vi "Export dat - C-V.vi"(8 "Error In":errorcluster, 9 "Workspace":path, 11 "C-V measurement":T1 {"CV properties"."V range" items=["10mV"=0.01, "100mV"=0.1, "1V"=1.0, "10V"=10.0]; "CV properties"."I range" items=["100nA"=-7.0, "1µA"=-6.0, "10µA"=-5.0, "100µA"=-4.0, "1mA"=-3.0, "10mA"=-2.0]}) -> (0 "Error Out":errorcluster)   [LabVIEW 2019]
doc: "Handles export of a C-V measurement to a .dat file, displays a GUI window"
uses:
  Type defs/CV measurement Type Def.ctl
  Type defs/CV properties Type Def.ctl
  <vilib>/Utility/sysdir.llb/System Directory Type.ctl
  <vilib>/Utility/file.llb/Write Delimited Spreadsheet (string).vi
  <vilib>/Utility/file.llb/Write Delimited Spreadsheet (DBL).vi
panel:
  out "String":string
  in  "Path":path caption="Export file as:"
  in  "Export":bool
  in  "Cancel":bool
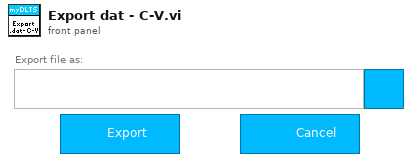
[diagram p1: front panel]
types:
  T1 = typedef "CV measurement Type Def.ctl" = cluster{"Name":string, "Comment":string, "Time":timestamp, "Folder":path, "CV properties":T2, "GUID":string}
  T2 = typedef "CV properties Type Def.ctl" = cluster{"T":dbl[unit], "Vstart":dbl[unit], "Vstop":dbl[unit], "Vpoints":dbl, "Precision":enum16{"Low (Fast)", "Normal", "High (Slow)"}, "Test signal":dbl[unit], "Auto I range":bool, "Test frequency":dbl[unit], "I range":dbl, "V range":dbl[unit], "Log mapping":bool, "Rel perm":dbl, "Area":dbl[unit]}
  T3 = enum32{"existing file", "new file", "new or existing file", "existing dir", "new dir", "new or existing dir", "existing file (use LLBs)", "new file (use LLBs)", "new or existing file (use LLBs)", "new or existing file or directory (use LLBs)", "existing dir (use LLBs)", "new dir (use LLBs)", "new or existing dir (use LLBs)", "existing file or dir", "new file or dir", "new or existing file or dir", "existing file or dir (use LLBs)", "new file or dir (use LLBs)"}
  T4 = typedef "System Directory Type.ctl" = i32
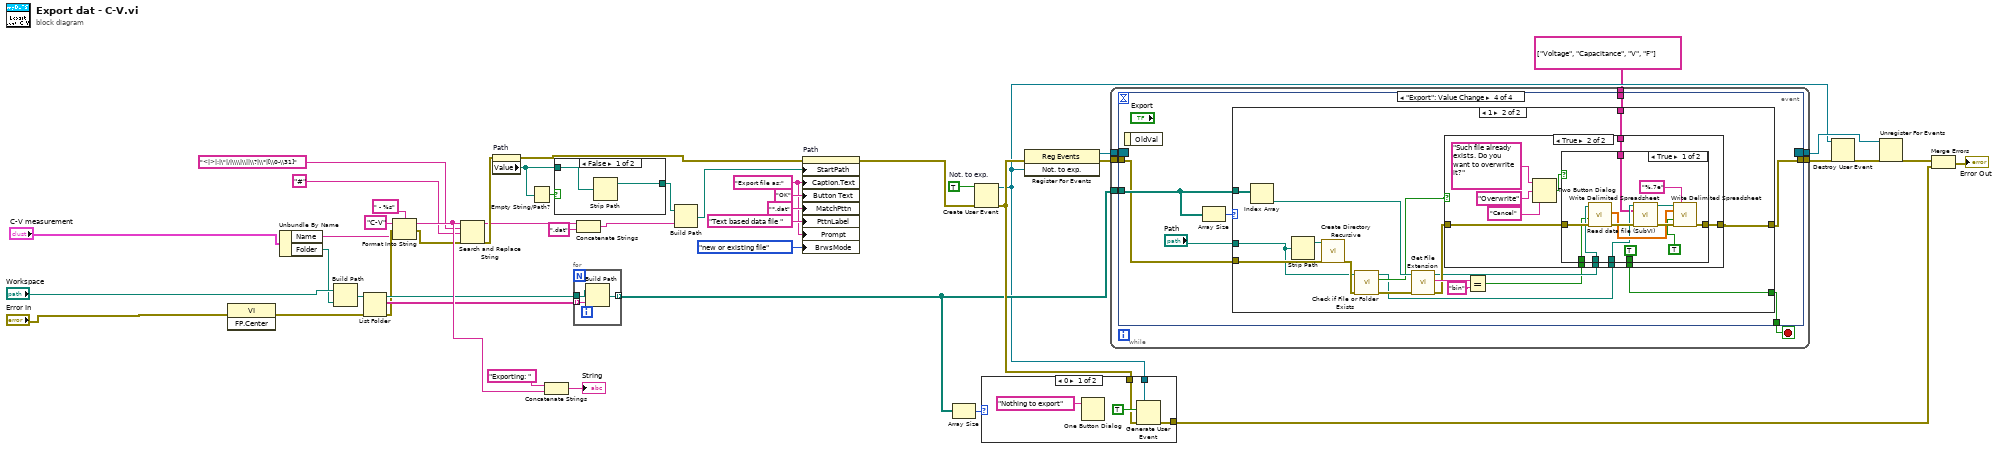
[diagram p0: block diagram]
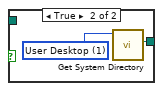
[diagram p2: hidden frame]
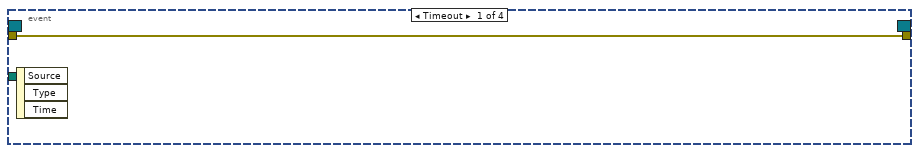
[diagram p4: hidden frame]
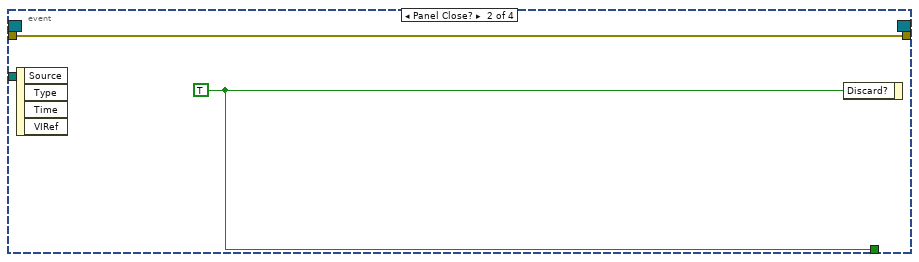
[diagram p5: hidden frame]
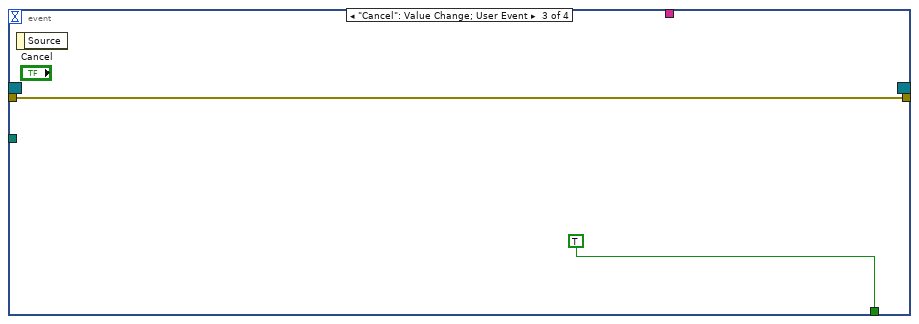
[diagram p6: hidden frame]
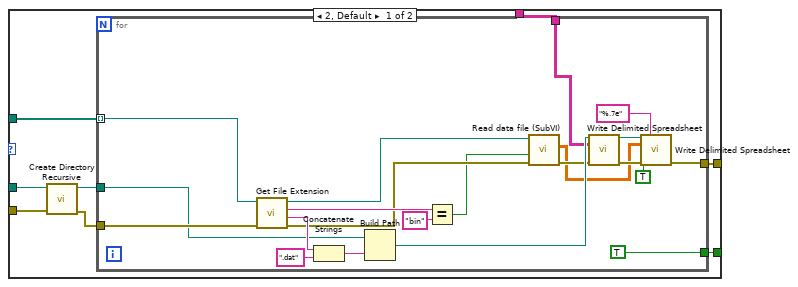
[diagram p7: hidden frame]
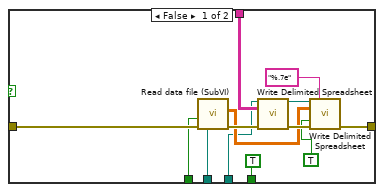
[diagram p8: hidden frame]
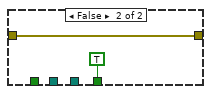
[diagram p9: hidden frame]
diagram:
  w15 = "Export file as:"
  w45 = TRUE  # Not. to exp.
  n1 = invoke class="VI" method="FP.Center"(error in="Error In") -> (error out=w2:errorcluster)  [unwired: 2 in, 2 out]
  n2 = Unbundle By Name("C-V measurement") -> ("Name"=w6:string, "Folder"=w20:path)
  n3 = Build Path(base path="Workspace", name or relative path=w20) -> (appended path=w13:path)
  n4 = List Folder(path=w13, error in=w2) -> (path out=w12:path, filenames=w19:string[], error out=w8:errorcluster)  [unwired: 2 in, 1 out]
  n5 = Format Into String(format string=" - %s", initial string="C-V", error in=w8, w6) -> (resulting string=w32:string, error out=w7:errorcluster)
  n6 = Search and Replace String(input string=w32, search string="<|>|:|\"|/|\\\\|\\||\\?|\\*|[\\0-\\31]", replace string="#" ("replace string (\"\")"), error in=w7) -> (result string=w5:string, error out=w9:errorcluster)  [unwired: 4 in, 2 out]
  n7 = property on="Path" class="Path"(error in=w9) -> (error out=w21:errorcluster, "Value"=w27:path)  [unwired: 1 in, 1 out]
  n8 = Empty String/Path?(string/path=w27) -> (empty?=w28:bool)
  n9 = Concatenate Strings("Exporting: " ("string"), w32) -> (→"String":string)
  n10 = case shown="False" w28 {
    tunnel: w27 -> [w49 _]
    tunnel: [w48 w50] -> w23
    frame False {
      n11 = Strip Path(path=w49) -> (stripped path=w48:path)  [unwired: 1 out]
    }
    frame True {
      w51 = T4 1 items=["User Home"=0, "User Desktop"=1, "User Documents"=2, "User Application Data"=3, "User Preferences"=4, "User Temporary"=5, "Public Documents"=6, "Public Application Data"=7, "Public Preferences"=8, "Public Cache"=13, "System Core Libraries"=9, "System Installed Libraries"=10, "Application Files"=11, "Boot Volume Root"=12] ("system directory type")
      n12 = call <vilib>:"Get System Directory.vi"("system directory type"=w51) -> ("system directory"=w50:path)  [unwired: 10 in]
    }
  }
  n13 = for {
    tunnel: w12 -> [w54]
    tunnel: [w53] -> w40 mode=indexing
    tunnel: w19 -> [w52] mode=indexing
    n14 = Build Path(base path=w54, name or relative path=w52) -> (appended path=w53:path)
  }
  n15 = Concatenate Strings(w5, ".dat" ("string")) -> (w10:string)
  n16 = Build Path(base path=w23, name or relative path=w10) -> (appended path=w22:path)
  n17 = property on="Path" class="Path"(error in=w21, "StartPath"=w22, "Caption.Text"=w15, "Button Text"="OK", "MatchPttn"="*.dat", "PttnLabel"="Text based data file ", "Prompt"=w15, "BrwsMode"=T3."new or existing file" ("Browse Options:Selection Mode")) -> (error out=w42:errorcluster)  [unwired: 1 in, 1 out]
  n18 = Array Size(array=w40) -> (size(s)=w46:i32)
  n19 = Create User Event(user event datatype=w45, error in=w42) -> (user event=w36:refnum<user-event>, error out=w41:errorcluster)
  n20 = case shown="0" w46 {
    tunnel: w36 -> [w58 _]
    tunnel: w41 -> [w56 w60]
    tunnel: [w55 w60] -> w33
    frame 0 {
      n21 = One Button Dialog(message="Nothing to export") -> ()  [unwired: 1 in, 1 out]
      n22 = Generate User Event(user event=w58, event data cluster=TRUE ("event data"), error in=w56) -> (error out=w55:errorcluster)  [unwired: 1 in, 1 out]
    }
    frame 1, Default {
    }
  }
  n23 = register-events(error in=w41, w36) -> (reference out=w43:refnum<event-registration>, error out=w44:errorcluster)  [unwired: 1 in]
  n24 = while {
    tunnel: w44 -> [w67]
    tunnel: [w66] -> w39
    tunnel: w40 -> [w64]
    tunnel: w43 -> [w63]
    tunnel: [w62] -> w37
    tunnel: string[][] [["Voltage", "Capacitance"], ["V", "F"]] ("2D data") -> [w61]
    stop <- w65 stop-if-true
    n25 = event shown="[3] \"Export\": Value Change" {
      selector: w63 -> [_ _ _ _]
      dyn-events: [_ _ _ _] -> w62
      timeout: _ -> [_ _ _ _]
      tunnel: w67 -> [w68 w69 w71 w77]
      tunnel: [w68 w69 w71 w76] -> w66
      tunnel: [_ w70 TRUE ("Discard?") w75] -> w65
      tunnel: w64 -> [_ _ _ w78]
      tunnel: w61 -> [_ _ _ w73]
      event Timeout {
        n26 = event-data() -> ()  [unwired: 1 in, 3 out]
      }
      event Panel Close? {
        w70 = TRUE ("Discard?")
        n27 = event-data() -> ()  [unwired: 1 in, 4 out]
        n28 = event-data("Discard?"=w70) -> ()  [unwired: 1 in, 1 out]
      }
      event "Cancel": Value Change; User Event {
        n29 = event-data() -> ()  [unwired: 1 in, 1 out]
      }
      event "Export": Value Change {
        n30 = event-data() -> ()  [unwired: 1 in, 1 out]
        n31 = Array Size(array=w78) -> (size(s)=w79:i32)
        n32 = case shown="1" w79 {
          tunnel: [w87 w112] -> w75
          tunnel: w77 -> [w84 w120]
          tunnel: w78 -> [w86 w119]
          tunnel: "Path" -> [w83 w117]
          tunnel: [w85 w116] -> w76
          tunnel: w73 -> [w80 w115]
          frame 2, Default {
            n33 = call <vilib>:"Create Directory Recursive.vi"("error in (no error)"=w84, "directory"=w83) -> ("error out"=w82:errorcluster, "directory copy"=w81:path)  [unwired: 3 in, 1 out]
            n34 = for {
              tunnel: [TRUE] -> w87
              tunnel: w86 -> [w105] mode=indexing
              tunnel: [w91] -> w85
              tunnel: w82 -> [w101]
              tunnel: w81 -> [w100]
              tunnel: w80 -> [w88]
              n35 = call <vilib>:"Get File Extension.vi"("error in (no error)"=w101, "file"=w105) -> ("error out"=w95:errorcluster, "filename without extension"=w103:string, "lowercase file extension"=w108:string, "dup file"=w96:path)  [unwired: 5 in, 1 out]
              n36 = Concatenate Strings(w103, ".dat" ("string")) -> (w104:string)
              n37 = Build Path(base path=w100, name or relative path=w104) -> (appended path=w93:path)
              n38 = Equal?(x=w108, y="bin") -> (x = y?=w94:bool)
              n39 = call "Read data file (SubVI).vi"("error in"=w95, "Binary"=w94, "file path in"=w96) -> ("error out"=w90:errorcluster, "2D data"=w89:dbl[][])  [unwired: 6 in, 1 out]
              n40 = call-poly <vilib>:"Write Delimited Spreadsheet.vi"("file path (dialog if empty)"=w93, "2D data"=w88, "error in (no error)"=w90) -> ("new file path (Not A Path if cancelled)"=w92:path, "error out"=w98:errorcluster)  [unwired: 11 in]
              n41 = call-poly <vilib>:"Write Delimited Spreadsheet.vi"("file path (dialog if empty)"=w92, "format (%.3f)"="%.7e", "2D data"=w89, "append to file? (new file:F)"=TRUE, "error in (no error)"=w98) -> ("error out"=w91:errorcluster)  [unwired: 9 in, 1 out]
            }
          }
          frame 1 {
            n42 = Index Array(array=w119) -> (element=w118:path)  [unwired: 1 in]
            n43 = Strip Path(path=w117) -> (stripped path=w122:path)  [unwired: 1 out]
            n44 = call <vilib>:"Create Directory Recursive.vi"("error in (no error)"=w120, "directory"=w122) -> ("error out"=w121:errorcluster)  [unwired: 3 in, 2 out]
            n45 = call <vilib>:"Check if File or Folder Exists.vi"("error in (no error)"=w121, "path"=w117) -> ("error out"=w123:errorcluster, "file or folder exists?"=w114:bool, "dup path"=w111:path)  [unwired: 7 in]
            n46 = call <vilib>:"Get File Extension.vi"("error in (no error)"=w123, "file"=w118) -> ("error out"=w113:errorcluster, "lowercase file extension"=w125:string, "dup file"=w110:path)  [unwired: 5 in, 2 out]
            n47 = Equal?(x=w125, y="bin") -> (x = y?=w109:bool)
            n48 = case shown="True" w114 {
              tunnel: [w131 w149] -> w116
              tunnel: [TRUE w148] -> w112
              tunnel: w113 -> [w129 w143]
              tunnel: w111 -> [w126 w142]
              tunnel: w110 -> [w127 w141]
              tunnel: w109 -> [w128 w140]
              tunnel: w115 -> [w130 w139]
              frame False {
                n49 = call "Read data file (SubVI).vi"("error in"=w129, "Binary"=w128, "file path in"=w127) -> ("error out"=w134:errorcluster, "2D data"=w133:dbl[][])  [unwired: 6 in, 1 out]
                n50 = call-poly <vilib>:"Write Delimited Spreadsheet.vi"("file path (dialog if empty)"=w126, "2D data"=w130, "error in (no error)"=w134) -> ("new file path (Not A Path if cancelled)"=w135:path, "error out"=w137:errorcluster)  [unwired: 11 in]
                n51 = call-poly <vilib>:"Write Delimited Spreadsheet.vi"("file path (dialog if empty)"=w135, "format (%.3f)"="%.7e", "2D data"=w133, "append to file? (new file:F)"=TRUE, "error in (no error)"=w137) -> ("error out"=w131:errorcluster)  [unwired: 9 in, 1 out]
              }
              frame True {
                n52 = Two Button Dialog(message="Such file already exists. Do you want to overwrite it?", 1:"Cancel" ("F button name (\"Cancel\")"), 2:"Overwrite" ("T button name (\"OK\")")) -> (T button?=w144:bool)
                n53 = case shown="True" w144 {
                  tunnel: [w155 w163] -> w149
                  tunnel: [TRUE TRUE] -> w148
                  tunnel: w143 -> [w156 w163]
                  tunnel: w142 -> [w154 _]
                  tunnel: w141 -> [w153 _]
                  tunnel: w140 -> [w152 _]
                  tunnel: w139 -> [w150 _]
                  frame True {
                    n54 = call "Read data file (SubVI).vi"("error in"=w156, "Binary"=w152, "file path in"=w153) -> ("error out"=w158:errorcluster, "2D data"=w157:dbl[][])  [unwired: 6 in, 1 out]
                    n55 = call-poly <vilib>:"Write Delimited Spreadsheet.vi"("file path (dialog if empty)"=w154, "2D data"=w150, "error in (no error)"=w158) -> ("new file path (Not A Path if cancelled)"=w159:path, "error out"=w161:errorcluster)  [unwired: 11 in]
                    n56 = call-poly <vilib>:"Write Delimited Spreadsheet.vi"("file path (dialog if empty)"=w159, "format (%.3f)"="%.7e", "2D data"=w157, "append to file? (new file:F)"=TRUE, "error in (no error)"=w161) -> ("error out"=w155:errorcluster)  [unwired: 9 in, 1 out]
                  }
                  frame False {
                  }
                }
              }
            }
          }
        }
      }
    }
  }
  n57 = Destroy User Event(user event=w36, error in=w39) -> (error out=w38:errorcluster)
  n58 = Unregister For Events(event registration refnum=w37, error in=w38) -> (error out=w35:errorcluster)
  n59 = Merge Errors(w35, w33) -> (→"Error Out":errorcluster)
